vi "svx_Write Excitations_Read Responses (DAQmx).vi"(0 "acquisition task":T1={"AI device settings"={"AI DAQmx TaskID"="", "response"=[{"AI physical channel"="Dev1/ai0", "AI channel settings"={"max value [V]"=10.0, "min value [V]"=-10.0, "terminal config"=10083, "DSA channel settings"={"coupling"=10045, "enable IEPE excitation"=FALSE, "IEPE current [mA]"=4.0}}}]}, "acquisition type"=enum."Finite", "measurement settings"={"AI sampling frequency"=51200.0, "AO sampling frequency"=51200.0, "AI block size"=0, "AO block Size"=0, "block duration [ms]"=100.0, "number of AI channels"=0, "device propagation delay [samples]"=0.0, "DUT propagation time [s]"=0.0}, "settling settings"={"settle time"=0.015599999576807022, "settle cycles"=5}, "integration settings"={"integration time"=0.015599999576807022, "integration cycles"=5}, "AO device settings"={"AO DAQmx taskID"="", "excitation"=[]}, "acquisition accounting"={"initial read size [samples]"=0, "read offset [samples]"=0, "read length [samples]"=0, "blocks to settle [samples]"=0, "min delay until transition [samples]"=0}, "frequency range"={"start frequency"=-1.0, "stop frequency"=-1.0}, "block type"=enum."Initialize", "source settings"={"signal type"=enum."Sine wave", "frequency"=0.0, "total amplitude"=0.0, "frequencies"=[1.0], "relative amplitudes"=[1.0], "offset"=1.0, "total amplitude list"=[1.0], "ramping rate"=0.0}, "chirp settings"={"amplitude"=0.0, "frequency range"={"start (Hz)"=20.0, "stop (Hz)"=20000.0, "frequency spacing"=enum."Logarithmic"}, "sampling info"={"Fs"=50000.0, "chirp duration [s]"=3.0}, "initial states"={"frequency [Hz]"=20.0, "phase [rad]"=0.0, "elapsed time [s]"=0.0}, "frequency slope"=0.0, "maximum harmonic"=0, "prefix len [samples]"={"integer"=0, "fractional"=0.0}}} {"chirp settings"."frequency slope" format="%.2f"; "chirp settings"."prefix len [samples]"."fractional" format="%.2p"; "chirp settings"."initial states"."elapsed time [s]" format="%.2f"; "chirp settings"."initial states"."phase [rad]" format="%.2f"; "chirp settings"."initial states"."frequency [Hz]" format="%.2f"; "chirp settings"."sampling info"."chirp duration [s]" format="%.2f"; "chirp settings"."sampling info"."Fs" format="%.2p"; "chirp settings"."frequency range"."stop (Hz)" format="%.2f"; "chirp settings"."frequency range"."start (Hz)" format="%.2f"; "chirp settings"."amplitude" format="%.2f"; "source settings"."total amplitude" format="%.2f"; "source settings"."relative amplitudes" format="%.2f"; "source settings"."frequencies" format="%.2f"; "source settings"."total amplitude list" format="%.2f"; "source settings"."ramping rate" format="%.4f"; "source settings"."offset" format="%.2f"; "source settings"."frequency" format="%.2f"; "frequency range"."stop frequency" format="%.2f"; "frequency range"."start frequency" format="%.2f"; "AO device settings"."excitation"."AO channel settings"."terminal config" items=["Default"=-1, "Differential"=10106, "Pseudodifferential"=12529]; "AI device settings"."response"."AI channel settings"."DSA channel settings"."IEPE current [mA]" min=0.0 max=20.0 format="%.1f"; "AI device settings"."response"."AI channel settings"."DSA channel settings"."coupling" items=["AC"=10045, "DC"=10050, "GND"=10066]; "AI device settings"."response"."AI channel settings"."min value [V]" format="%.2f"; "AI device settings"."response"."AI channel settings"."terminal config" items=["Default"=-1, "RSE"=10083, "NRSE"=10078, "Differential"=10106, "Pseudodifferential"=12529]; "AI device settings"."response"."AI channel settings"."max value [V]" format="%.2f"; "integration settings"."integration time" format="%.2p"; "settling settings"."settle time" format="%.2p"; "measurement settings"."DUT propagation time [s]" format="%.2f"; "measurement settings"."AO sampling frequency" format="%.2f"; "measurement settings"."AI sampling frequency" format="%.2f"}, 11 "error in (no error)":errorcluster, 12 "iteration":i32) -> (3 "status":T5, 4 "acquisition task":T1={"AI device settings"={"AI DAQmx TaskID"="", "response"=[{"AI physical channel"="Dev1/ai0", "AI channel settings"={"max value [V]"=10.0, "min value [V]"=-10.0, "terminal config"=10083, "DSA channel settings"={"coupling"=10045, "enable IEPE excitation"=FALSE, "IEPE current [mA]"=4.0}}}]}, "acquisition type"=enum."Finite", "measurement settings"={"AI sampling frequency"=51200.0, "AO sampling frequency"=51200.0, "AI block size"=0, "AO block Size"=0, "block duration [ms]"=100.0, "number of AI channels"=0, "device propagation delay [samples]"=0.0, "DUT propagation time [s]"=0.0}, "settling settings"={"settle time"=0.015599999576807022, "settle cycles"=5}, "integration settings"={"integration time"=0.015599999576807022, "integration cycles"=5}, "AO device settings"={"AO DAQmx taskID"="", "excitation"=[]}, "acquisition accounting"={"initial read size [samples]"=0, "read offset [samples]"=0, "read length [samples]"=0, "blocks to settle [samples]"=0, "min delay until transition [samples]"=0}, "frequency range"={"start frequency"=-1.0, "stop frequency"=-1.0}, "block type"=enum."Initialize", "source settings"={"signal type"=enum."Sine wave", "frequency"=0.0, "total amplitude"=0.0, "frequencies"=[1.0], "relative amplitudes"=[1.0], "offset"=1.0, "total amplitude list"=[1.0], "ramping rate"=0.0}, "chirp settings"={"amplitude"=0.0, "frequency range"={"start (Hz)"=20.0, "stop (Hz)"=20000.0, "frequency spacing"=enum."Logarithmic"}, "sampling info"={"Fs"=50000.0, "chirp duration [s]"=3.0}, "initial states"={"frequency [Hz]"=20.0, "phase [rad]"=0.0, "elapsed time [s]"=0.0}, "frequency slope"=0.0, "maximum harmonic"=0, "prefix len [samples]"={"integer"=0, "fractional"=0.0}}} {"chirp settings"."frequency slope" format="%.2f"; "chirp settings"."prefix len [samples]"."fractional" format="%.2p"; "chirp settings"."initial states"."elapsed time [s]" format="%.2f"; "chirp settings"."initial states"."phase [rad]" format="%.2f"; "chirp settings"."initial states"."frequency [Hz]" format="%.2f"; "chirp settings"."sampling info"."chirp duration [s]" format="%.2f"; "chirp settings"."sampling info"."Fs" format="%.2p"; "chirp settings"."frequency range"."stop (Hz)" format="%.2f"; "chirp settings"."frequency range"."start (Hz)" format="%.2f"; "chirp settings"."amplitude" format="%.2f"; "source settings"."total amplitude" format="%.2f"; "source settings"."relative amplitudes" format="%.2f"; "source settings"."frequencies" format="%.2f"; "source settings"."total amplitude list" format="%.2f"; "source settings"."ramping rate" format="%.4f"; "source settings"."offset" format="%.2f"; "source settings"."frequency" format="%.2f"; "frequency range"."stop frequency" format="%.2f"; "frequency range"."start frequency" format="%.2f"; "AO device settings"."excitation"."AO channel settings"."terminal config" items=["Default"=-1, "Differential"=10106, "Pseudodifferential"=12529]; "AI device settings"."response"."AI channel settings"."DSA channel settings"."IEPE current [mA]" min=0.0 max=20.0 format="%.1f"; "AI device settings"."response"."AI channel settings"."DSA channel settings"."coupling" items=["AC"=10045, "DC"=10050, "GND"=10066]; "AI device settings"."response"."AI channel settings"."min value [V]" format="%.2f"; "AI device settings"."response"."AI channel settings"."terminal config" items=["Default"=-1, "RSE"=10083, "NRSE"=10078, "Differential"=10106, "Pseudodifferential"=12529]; "AI device settings"."response"."AI channel settings"."max value [V]" format="%.2f"; "integration settings"."integration time" format="%.2p"; "settling settings"."settle time" format="%.2p"; "measurement settings"."DUT propagation time [s]" format="%.2f"; "measurement settings"."AO sampling frequency" format="%.2f"; "measurement settings"."AI sampling frequency" format="%.2f"}, 6 "data to process":waveform(dbl)[](array[waveform]), 8 "new data to process":bool, 10 "finished":bool, 13 "generated excitations":waveform(dbl)[](array[waveform]), 14 "all acquired data":waveform(dbl)[](array[waveform]), 15 "error out":errorcluster)   [LabVIEW 2017]
doc: "This example VI controls both the analog input and analog output after an audio measurement has begun. \n\nThis VI should be called after <B>SVXMPL_Start.vi</B>. If the <B>acquisition type</B> is defined as \"Finite\" in <B>SVXMPL_Initialize.vi</B>, you generally will make a single call to <B>SVXMPL_Write Excitations_Read Responses</B>. If you are using another aquisition type, you will generally place <B>SVXMPL_Write Excitations_Read Responses</B> in a loop.\n\nIf you are using this VI in a loop, be sure to wire the loop iteration counter to the <B>iteration</B> input. \n\nThe <B>status</B> indicator returns the number of scans read on input, the number of scans generated on output, and the input scan backlog.\n\nThe <B>new data to process</B> indicator is a boolean value indicating whether the data that has been acquired should be processed as part of the audio measurement. This indicator will return FALSE if the DUT is still settling, for example. SVT audio analysis functions may be peformed in a CASE structure controlled by this boolean to guarantee that you process only useful data.\n\n<B>data to process</B> returns data that should be analyzed. If the <B>new data to process</B> indicator returns a FALSE value, the <B>data to process</B> will return an empty array.\n\n<B>all acquired data</B> returns all data points, whether or not these points are intended to be analyzed. This can be useful, for example, in determining whether the DUT settling parameters you have specified are accurate.\n\n<B>generated excitations</B> returns the waveform date used to produce the stimulus signal."
uses:
  <vilib>/addons/Sound and Vibration/Example Support/Audio/DAQmx/svx_Acquisition Task (DAQmx).ctl
  <vilib>/addons/_NISVFA/_Shared subVIs/Controls/svc_Channel Settings.ctl
  <vilib>/addons/_NISVFA/_Shared subVIs/Controls/svc_DSA Channel Settings.ctl
  <vilib>/addons/_NISVFA/_Generation/subVIs/sv_Chirp Settings.ctl
  <vilib>/addons/_NISVFA/_Generation/SoundVib_Generation.lvlib
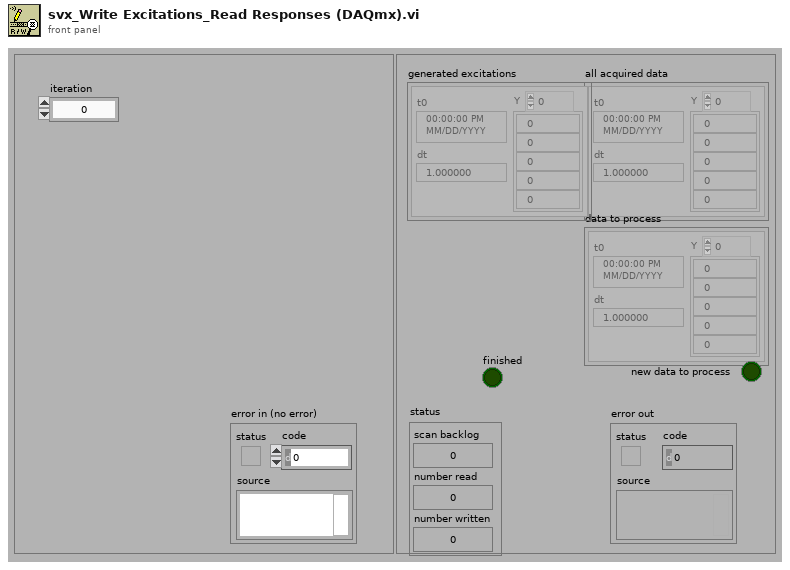
[diagram p1: front panel]
types:
  T1 = typedef "svx_Acquisition Task (DAQmx).ctl" = cluster{"AI device settings":cluster{"AI DAQmx TaskID":refnum<k21>, "response":cluster{"AI physical channel":tag, "AI channel settings":T2}[]}, "acquisition type":enum16{"Finite", "Averaged", "Settled", "Amplitude Sweep", "Stepped Frequency Sweep", "Continuous Frequency Sweep"}, "measurement settings":cluster{"AI sampling frequency":dbl, "AO sampling frequency":dbl, "AI block size":i32, "AO block Size":i32, "block duration [ms]":dbl, "number of AI channels":i32, "device propagation delay [samples]":dbl, "DUT propagation time [s]":dbl}, "settling settings":cluster{"settle time":dbl, "settle cycles":i32}, "integration settings":cluster{"integration time":dbl, "integration cycles":i32}, "AO device settings":cluster{"AO DAQmx taskID":refnum<k21>, "excitation":cluster{"AO physical channel":tag, "AO channel settings":cluster{"maximum value (10 V)":dbl, "minimum value (10 V)":dbl, "terminal config":i32}}[]}, "acquisition accounting":cluster{"initial read size [samples]":i32, "read offset [samples]":i32, "read length [samples]":i32, "blocks to settle [samples]":i32, "min delay until transition [samples]":i32}, "frequency range":cluster{"start frequency":dbl, "stop frequency":dbl}, "block type":enum16{"Initialize", "Settle", "Integrate"}, "source settings":cluster{"signal type":enum16{"Sine wave", "Dual tone (IMD)", "Multitone", "Chirp", "Frequency flat chirp", "Uniform white noise", "Gaussian white noise", "Pink noise", "PRN", "Continuous swept-sine"}, "frequency":dbl, "total amplitude":dbl, "frequencies":dbl[], "relative amplitudes":dbl[], "offset":dbl, "total amplitude list":dbl[], "ramping rate":dbl}, "chirp settings":T4}
  T2 = typedef "svc_Channel Settings.ctl" = cluster{"max value [V]":dbl, "min value [V]":dbl, "terminal config":i32, "DSA channel settings":T3}
  T3 = typedef "svc_DSA Channel Settings.ctl" = cluster{"coupling":i32, "enable IEPE excitation":bool, "IEPE current [mA]":dbl}
  T4 = typedef "SoundVib_Generation.lvlib/sv_Chirp Settings.ctl" = cluster{"amplitude":dbl, "frequency range":cluster{"start (Hz)":dbl, "stop (Hz)":dbl, "frequency spacing":enum16{"Linear", "Logarithmic"}}, "sampling info":cluster{"Fs":dbl, "chirp duration [s]":dbl}, "initial states":cluster{"frequency [Hz]":dbl, "phase [rad]":dbl, "elapsed time [s]":dbl}, "frequency slope":dbl, "maximum harmonic":i32, "prefix len [samples]":cluster{"integer":u32, "fractional":dbl}}
  T5 = cluster{"scan backlog":u32, "number read":i32, "number written":i32}
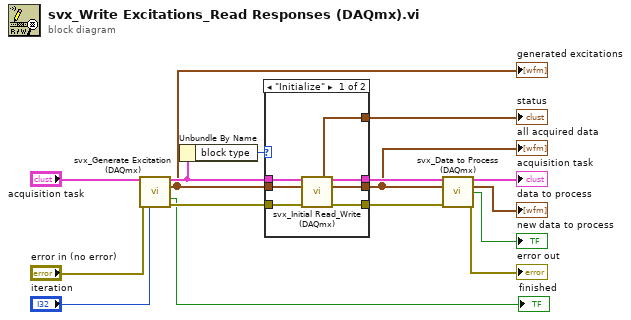
[diagram p0: block diagram]
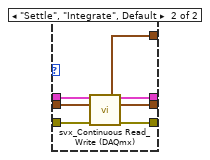
[diagram p2: hidden frame]
diagram:
  n1 = call <vilib>:"svx_Generate Excitation (DAQmx).vi"("acquisition task"="acquisition task", "error in (no error)"="error in (no error)", "Iteration"="iteration") -> ("acquisition task out"=w11:T1, "waveform excitation"=w2:waveform(dbl)[], "end reached"=→"finished":bool, "error out"=w13:errorcluster)  [unwired: 9 in]
  "generated excitations" <- w2
  n2 = Unbundle By Name(w11) -> ("block type"=w15:enum16{"Initialize", "Settle", "Integrate"})
  n3 = case shown="\"Initialize\"" w15 {
    tunnel: [w18 w24] -> w7
    tunnel: w13 -> [w17 w25]
    tunnel: w11 -> [w23 w30]
    tunnel: [w22 w29] -> w9
    tunnel: w2 -> [w21 w28]
    tunnel: [w20 w27] -> w4
    tunnel: [w19 w26] -> w16
    frame "Initialize" {
      n4 = call <vilib>:"svx_Initial Read_Write (DAQmx).vi"("acquisition task in"=w23, "waveform excitation"=w21, "error in (no error)"=w17) -> ("status"=w19:T5, "acquisition task out"=w22:T1, "waveform data"=w20:waveform(dbl)[], "error out"=w18:errorcluster)  [unwired: 8 in, 1 out]
    }
    frame "Settle", "Integrate", Default {
      n5 = call <vilib>:"svx_Continuous Read_Write (DAQmx).vi"("acquisition task in"=w30, "waveform excitations"=w28, "error in (no error)"=w25) -> ("status"=w26:T5, "acquisition task out"=w29:T1, "waveform responses"=w27:waveform(dbl)[], "error out"=w24:errorcluster)  [unwired: 9 in]
    }
  }
  "all acquired data" <- w4
  "status" <- w16
  n6 = call <vilib>:"svx_Data to Process (DAQmx).vi"("acquisition task"=w9, "waveform data"=w4, "error in (no error)"=w7) -> ("acquisition task"=→"acquisition task":T1, "data to process"=→"data to process":waveform(dbl)[], "new data to process"=→"new data to process":bool, "error out"=→"error out":errorcluster)  [unwired: 9 in]
